vi "ExposeBindParameter.vi"(6 "Bind Direction":T1=enum."Bidrectional", 7 "Val Change EV":refnum<k27>, 9 "Name (empty)":string, 10 "Value":variant, 11 "Expose Info":T2) -> ()   [LabVIEW 2017]
uses:
  Core/ExposeInfo.ctl
  C:/Code/CMCryoSysCode/Expose/COM/CSCom/CSCom/bin/Release/CSCom.dll
  COM/CSCom/CSCom/bin/Release/CSCom.dll
  ExposeParameterBindingType.ctl
  ExposeParameterBindingData.ctl
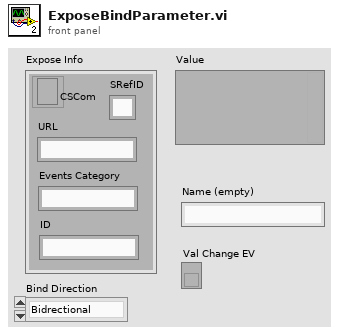
[diagram p1: front panel]
types:
  T1 = typedef "ExposeParameterBindingType.ctl" = enum16{"ToRemote", "FromRemote", "Bidrectional"}
  T2 = typedef "ExposeInfo.ctl" = cluster{"CSCom":refnum<k24>, "URL":string, "Events Category":string, "ID":string, "SRefID":string}
  T3 = typedef "ExposeDataType.ctl" = cluster{"Values":variant, "ParameterBindingInfo":variant}
  T4 = typedef "ExposeParameterBindingData.ctl" = cluster{"Val Change EV":refnum<k27>, "Bind Direction":T1, "Ignore Next\nUpdate Count":i32}
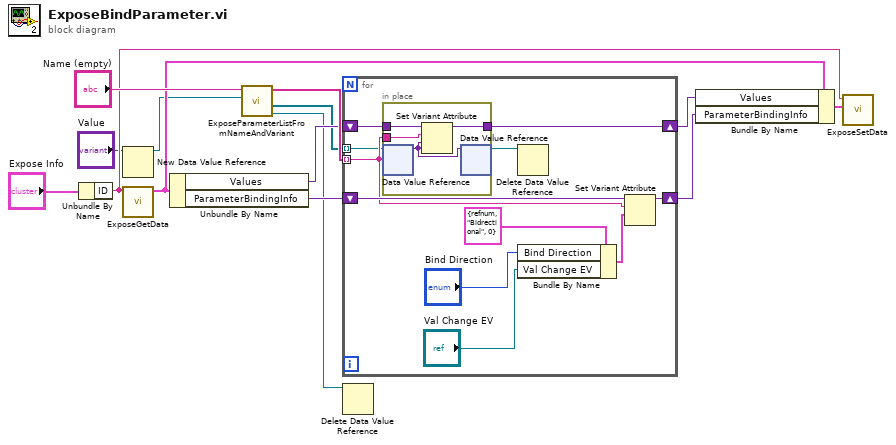
[diagram p0: block diagram]
diagram:
  n1 = Unbundle By Name("Expose Info") -> ("ID"=w11:string)
  n2 = New Data Value Reference(data value="Value") -> (data value reference=w3:refnum<data-value>)  [unwired: 1 in, 1 out]
  n3 = call "ExposeGetData.vi"("ExposeID"=w11) -> ("ExposeDataType"=w6:T3)  [unwired: 9 in, 1 out]
  n4 = Unbundle By Name(w6) -> ("Values"=w10:variant, "ParameterBindingInfo"=w9:variant)
  n5 = call "ExposeParameterListFromNameAndVariant.vi"("Value Reference In"=w3, "Name (empty)"="Name (empty)") -> ("Value Reference Out"=w1:refnum<data-value>, "Parmaeter Refs"=w2:refnum<data-value>[], "Parameter names"=w12:string[])  [unwired: 7 in]
  n6 = for {
    tunnel: w12 -> [w18] mode=indexing
    shift-right: [w25] -> w8
    shift-left: w10 -> [w21]
    shift-right: [w19] -> w7
    shift-left: w9 -> [w20]
    tunnel: w2 -> [w16] mode=indexing
    n7 = in-place {
      in-place-border: [w29] -> w25
      in-place-border: w21 -> [w28]
      in-place-border: w18 -> [w27]
      n8 = in-place-dvr #1(w16) -> (w26:variant)  [unwired: 1 out]
      n9 = Set Variant Attribute(Variant=w28, name=w27, value=w26) -> (Variant out=w29:variant)  [unwired: 1 in, 2 out]
      n10 = in-place-dvr #1(w26) -> (w15:refnum<data-value>)  [unwired: 1 out]
    }
    n11 = Delete Data Value Reference(data value reference=w15) -> ()  [unwired: 1 in, 2 out]
    n12 = Bundle By Name(cluster=T4 {"Val Change EV"=refnum, "Bind Direction"=enum."Bidrectional", "Ignore Next\nUpdate Count"=0} ("ExposeParmeterBindingData"), "Bind Direction"="Bind Direction", "Val Change EV"="Val Change EV") -> (w17:T4)
    n13 = Set Variant Attribute(Variant=w20, name=w18, value=w17) -> (Variant out=w19:variant)  [unwired: 1 in, 2 out]
  }
  n14 = Delete Data Value Reference(data value reference=w1) -> ()  [unwired: 1 in, 2 out]
  n15 = Bundle By Name(cluster=w6, "Values"=w8, "ParameterBindingInfo"=w7) -> (w5:T3)
  n16 = call "ExposeSetData.vi"("ExposeDataType"=w5, "ExposeID"=w11) -> ()  [unwired: 10 in]
